vi "PhotonTargetModel_New_RectPlanar.vi"(9 "Height Meters":dbl, 11 "Width Meters":dbl) -> (3 "PhotonTargetModel":T1 {"Vertices"."Z" format="%14.3f"; "Vertices"."Y" format="%14.3f"; "Vertices"."X" format="%14.3f"})   [LabVIEW 2019, in "PhotonVisionLib.lvlib"]
doc: "Creates a rectangular, planar target model given the width and height. The model has four vertices:\n \n - Point 0: [0, -width/2, -height/2]\n - Point 1: [0, width/2, -height/2]\n - Point 2: [0, width/2, height/2]\n - Point 3: [0, -width/2, height/2]\n\nInputs:\n - widthMeters - double - Width (meters)\n - HeightMeters - double - Height (meters)\n\nOutputs:\n - TargetModel - cluster - created target model"
uses:
  PhotonVisionLib.lvlib
  TypeDef/PhotonTargetModel.ctl
  <vilib>/Rock Robotics/WPI/ThirdParty/JAS_Junk/TrajLib/TypeDef/TRANSLATION3D.ctl
  <vilib>/Rock Robotics/WPI/ThirdParty/JAS_Junk/TrajLib/Trajectory_Library.lvlib
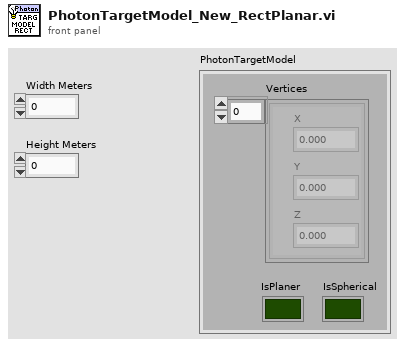
[diagram p1: front panel]
types:
  T1 = typedef "PhotonVisionLib.lvlib/PhotonTargetModel.ctl" = cluster{"Vertices":T2[], "IsPlaner":bool, "IsSpherical":bool}
  T2 = typedef "Trajectory_Library.lvlib/TRANSLATION3D.ctl" = cluster{"X":dbl, "Y":dbl, "Z":dbl}
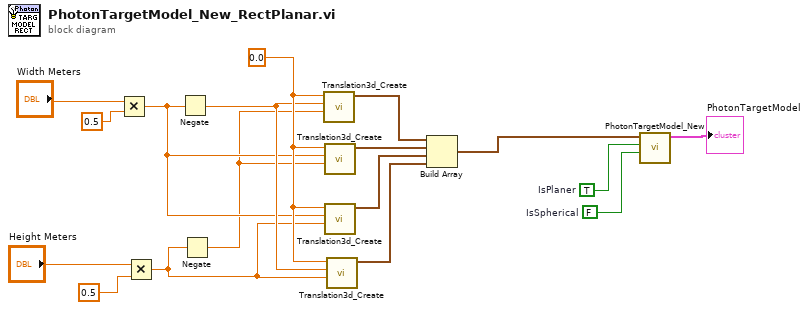
[diagram p0: block diagram]
diagram:
  w5 = 0.0 ("X")
  w6 = TRUE  # IsPlaner
  w7 = FALSE  # IsSpherical
  n1 = Multiply(x="Width Meters", y=0.5) -> (x*y=w3:dbl)
  n2 = Multiply(x="Height Meters", y=0.5) -> (x*y=w1:dbl)
  n3 = Negate(x=w3) -> (-x=w4:dbl)
  n4 = Negate(x=w1) -> (-x=w2:dbl)
  n5 = call <vilib>:"Translation3d_Create.vi"("Z"=w2, "Y"=w4, "X"=w5) -> ("TRANSLATION3D"=w13:T2)  [unwired: 8 in]
  n6 = call <vilib>:"Translation3d_Create.vi"("Z"=w2, "Y"=w3, "X"=w5) -> ("TRANSLATION3D"=w12:T2)  [unwired: 8 in]
  n7 = call <vilib>:"Translation3d_Create.vi"("Z"=w1, "Y"=w3, "X"=w5) -> ("TRANSLATION3D"=w11:T2)  [unwired: 8 in]
  n8 = call <vilib>:"Translation3d_Create.vi"("Z"=w1, "Y"=w4, "X"=w5) -> ("TRANSLATION3D"=w10:T2)  [unwired: 8 in]
  n9 = Build Array(w13, w12, w11, w10) -> (w9:T2[])
  n10 = call "PhotonTargetModel_New.vi"("IsSpherical"=w7, "IsPlaner"=w6, "Vertices"=w9) -> ("PhotonTargetModel"=→"PhotonTargetModel":T1)  [unwired: 8 in]
